vi "data UI ws.vi"() -> ()   [LabVIEW 2018]
uses:
  controls/test data.ctl
  controls/test.ctl
panel:
  in  "Test":T1=enum."phase R UV mOhm"
  out "Array":string[](array[string])
  out "Data":T2 {"UW - VW VDC" format="%.2g"; "UV - VW VCD" format="%.2g"; "UV - UW VDC" format="%.2g"; "UW - VW L uH" format="%.2g"; "UV - VW L uH" format="%.2g"; "UV - UW L uH" format="%.2g"; "UW - VW mOhm" format="%.2g"; "UV - VW mOhm" format="%.2g"; "UV - UW mOhm" format="%.2g"; "back EMF VW VDC" format="%.2g"; "back EMF UW VDC" format="%.2g"; "back EMF UV VDC" format="%.2g"; "phase L VW uH" format="%.2g"; "phase L UW uH" format="%.2g"; "phase L UV uH" format="%.2g"; "phase R VW mOhm" format="%.2g"; "phase R UW mOhm" format="%.2g"; "phase R UV mOhm" format="%.2g"}
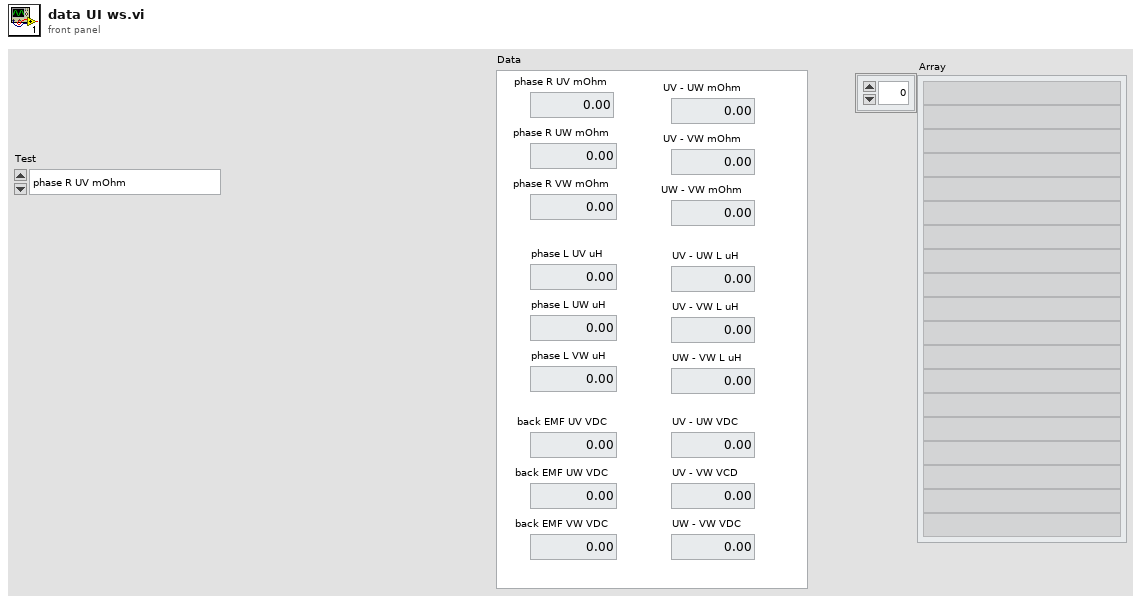
[diagram p1: front panel]
types:
  T1 = typedef "test.ctl" = enum16{"init", "default", "exit", "phase R UV mOhm", "phase R UW mOhm", "phase R VW mOhm", "phase L UV uH", "phase L UW uH", "phase L VW uH", "back EMF UV VDC", "back EMF UW VDC", "back EMF VW VDC", "UV - UW mOhm", "UV - VW mOhm", "UW - VW mOhm", "UV - UW L uH", "UV - VW L uH", "UW - VW L uH", "UV - UW VDC", "UV - VW VCD", "UW - VW VDC", "plot data", "save data", ""}
  T2 = typedef "test data.ctl" = cluster{"phase R UV mOhm":dbl, "phase R UW mOhm":dbl, "phase R VW mOhm":dbl, "phase L UV uH":dbl, "phase L UW uH":dbl, "phase L VW uH":dbl, "back EMF UV VDC":dbl, "back EMF UW VDC":dbl, "back EMF VW VDC":dbl, "UV - UW mOhm":dbl, "UV - VW mOhm":dbl, "UW - VW mOhm":dbl, "UV - UW L uH":dbl, "UV - VW L uH":dbl, "UW - VW L uH":dbl, "UV - UW VDC":dbl, "UV - VW VCD":dbl, "UW - VW VDC":dbl}
  T3 = enum8{"Enabled", "Disabled", "Disabled and Grayed Out"}
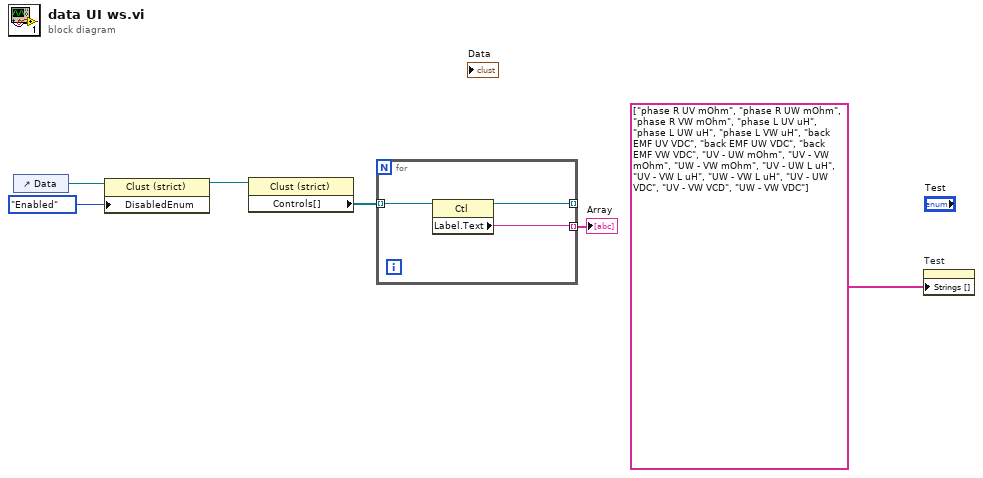
[diagram p0: block diagram]
diagram:
  n1 = control-ref of="Data"() -> (w6:refnum<vi>)
  n2 = property class="Clust (strict)"(reference=w6, "DisabledEnum"=T3."Enabled" ("Disabled")) -> (reference out=w4:refnum<vi>)  [unwired: 1 in, 1 out]
  n3 = property class="Clust (strict)"(reference=w4) -> ("Controls[]"=w3:refnum<vi>[])  [unwired: 1 in, 2 out]
  n4 = for {
    tunnel: w3 -> [w9] mode=indexing
    tunnel: [w8] -> w2 mode=indexing
    tunnel: [w7] -> _ mode=indexing
    n5 = property class="Ctl"(reference=w9) -> (reference out=w7:refnum<vi>, "Label.Text"=w8:string)  [unwired: 1 in, 1 out]
  }
  "Array" <- w2
  n6 = property on="Test" class="Enum (strict)"("Strings []"=string[] ["phase R UV mOhm", "phase R UW mOhm", "phase R VW mOhm", "phase L UV uH", "phase L UW uH", "phase L VW uH", "back EMF UV VDC", "back EMF UW VDC", "back EMF VW VDC", "UV - UW mOhm", "UV - VW mOhm", "UW - VW mOhm", "UV - UW L uH", "UV - VW L uH", "UW - VW L uH", "UV - UW VDC", "UV - VW VCD", "UW - VW VDC"] ("Array 2")) -> ()  [unwired: 2 in, 2 out]
